vi "Configure Standard Waveform.vi"(0 "VISA resource name":refnum<visa-resource-name>, 1 "Waveform Function (0: Sine)":u16(ring) items=["Sine", "Square", "Ramp", "DC", "Pulse", "Arb"], 2 "Channel (1:Channel 1)":i32(ring)=1 items=["Channel 1"=1, "Channel 2"=2], 5 "Amplitude (1.0 Vpp)":dbl=1.0 format="%#.3f", 7 "Frequency (1000 Hz)":dbl=1000.0 format="%#.6g", 9 "DC Offset (0.00 V)":dbl, 11 "error in (no error)":errorcluster, 12 "Phase (0.0 degrees)":dbl=0.002 min=-360.0 max=360.0 format="%#.1g") -> (4 "VISA resource name out":refnum<visa-resource-name>, 15 "error out":errorcluster)   [LabVIEW 2019, in "Siglent SDG X Series.lvlib"]
doc: "Selects the waveform shape, frequency, amplitude, offset, and phase for standard waveforms (including Sine, Square, Ramp, Pulse, DC and Arb).\n\nNotes: \nTo configure other parameters for pulse waveforms please run the Configure Pulse VI. \nTo configure noise waveform please run the Configure Noise VI.\nTo configure other parameters for arbitrary waveforms please run the Create Arbitrary Waveform. \nTo configure PRBS waveform please run the Configure PRBS Waveform VI."
uses:
  Siglent SDG X Series.lvlib
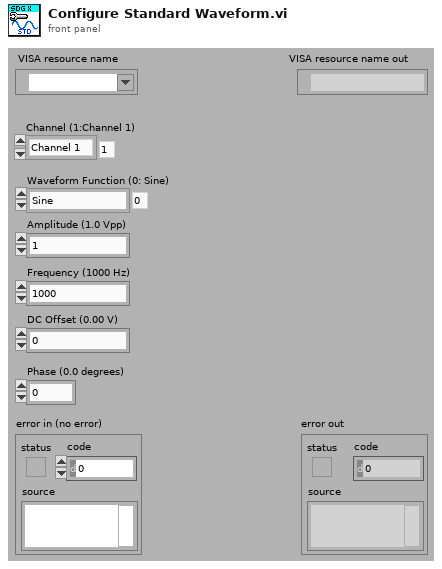
[diagram p1: front panel]
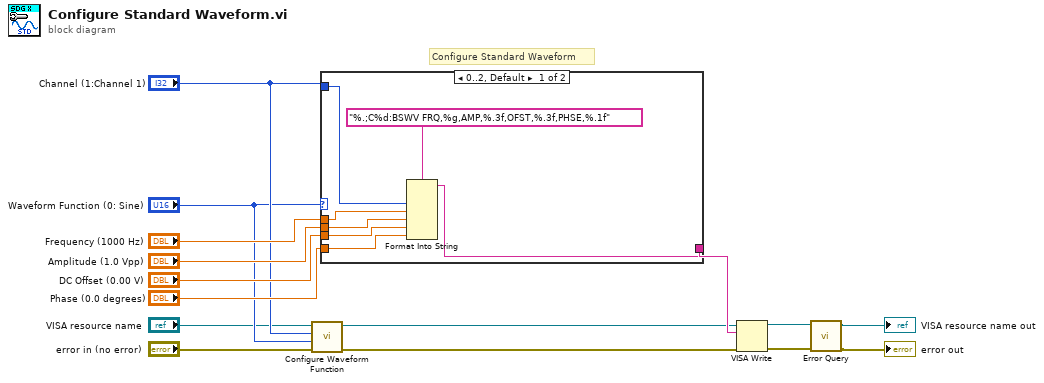
[diagram p0: block diagram]
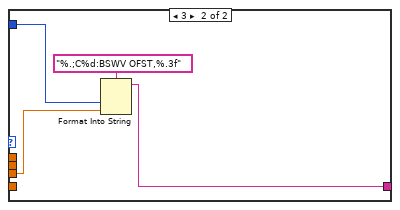
[diagram p2: hidden frame]
diagram:
  # "Configure Standard Waveform"
  n1 = call "Configure Waveform Function.vi"("error in (no error)"="error in (no error)", "Waveform Function (0: Sine)"="Waveform Function (0: Sine)", "Channel (1:Channel 1)"="Channel (1:Channel 1)", "VISA resource name"="VISA resource name") -> ("error out"=w1:errorcluster, "VISA resource name out"=w2:refnum<visa-resource-name>)  [unwired: 6 in]
  n2 = case shown="0..2, Default" "Waveform Function (0: Sine)" {
    tunnel: [w21 w23] -> w15
    tunnel: "Phase (0.0 degrees)" -> [w16 _]
    tunnel: "DC Offset (0.00 V)" -> [w17 w24]
    tunnel: "Amplitude (1.0 Vpp)" -> [w18 _]
    tunnel: "Frequency (1000 Hz)" -> [w19 _]
    tunnel: "Channel (1:Channel 1)" -> [w20 w25]
    frame 0..2, Default {
      n3 = Format Into String(format string="%.;C%d:BSWV FRQ,%g,AMP,%.3f,OFST,%.3f,PHSE,%.1f", w20, w19, w18, w17, w16) -> (resulting string=w21:string)  [unwired: 2 in, 1 out]
    }
    frame 3 {
      n4 = Format Into String(format string="%.;C%d:BSWV OFST,%.3f", w25, w24) -> (resulting string=w23:string)  [unwired: 2 in, 1 out]
    }
  }
  n5 = VISA Write(VISA resource name=w2, write buffer=w15, error in (no error)=w1) -> (VISA resource name out=w10:refnum<visa-resource-name>, error out=w9:errorcluster)  [unwired: 1 out]
  n6 = call "Error Query.vi"("error in (no error)"=w9, "VISA resource name"=w10) -> ("error out"=→"error out":errorcluster, "VISA resource name out"=→"VISA resource name out":refnum<visa-resource-name>)  [unwired: 6 in, 2 out]
